vi "MeasuredObj_set.vi"(8 "error in (no error)":errorcluster, 11 "MeasuredObjects":T1(array[cluster])) -> (0 "error out":errorcluster)   [LabVIEW 2009, in "NetworkVarTarget.lvlib"]
uses:
  NetworkVarTarget.lvlib
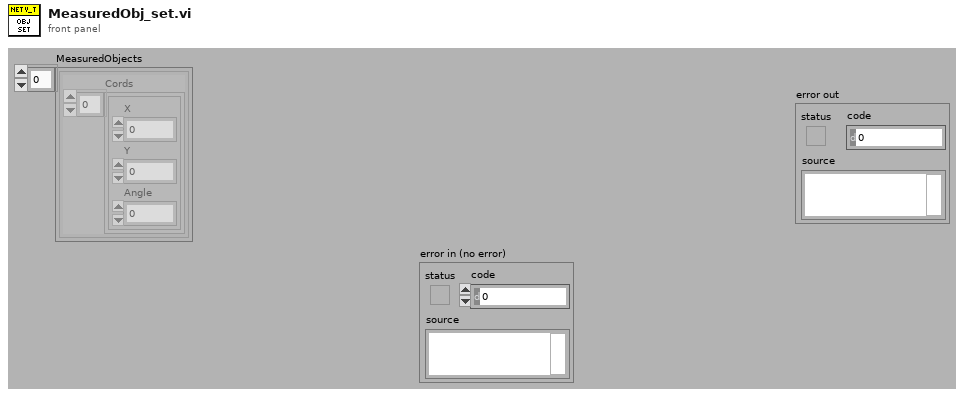
[diagram p1: front panel]
types:
  T1 = cluster{"Cords":cluster{"X":dbl, "Y":dbl, "Angle":dbl}[]}[]
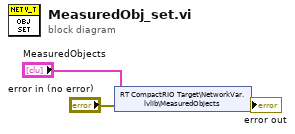
[diagram p0: block diagram]
diagram:
  n1 = shared-variable "RT CompactRIO Target\\NetworkVar.lvlib\\MeasuredObjects"("MeasuredObjects", error in="error in (no error)") -> (error out=→"error out":errorcluster)
